vi "Main.vi"(7 "sweep rate, /min":dbl=0.2, 8 "sweep to:":dbl=4.0, 9 "sweep":T8(radio)=enum."2636a_smub") -> ()   [LabVIEW 2021] (continued)
                      n3296 = local read "SR830 1 addr"() -> (w4460:u8)
                      n3297 = Number To Decimal String(number=w4460) -> (decimal integer string=w4459:string)  [unwired: 1 in]
                      n3298 = GPIB Write(0:w4459, 1:"OUTR?1") -> (6:w4465:errorcluster)  [unwired: 3 in, 1 out]
                      n3299 = GPIB Read(0:w4459, 1:3200, 3:w4465) -> (5:w4463:string)  [unwired: 2 in, 2 out]
                      n3300 = Fract/Exp String To Number(string=w4463) -> (number=w4462:dbl)  [unwired: 3 in, 1 out]
                      n3301 = Build Array (concatenate)(w4467, w4462) -> (w4466:dbl[])
                    }
                  }
                  n3302 = property on="data" class="Arr (strict)"("Value"=w4457) -> ()  [unwired: 2 in, 2 out]
                }
                frame #1 {
                  # "check if out-of-phase\nsignal on lock-in 1 \nis to be measured"
                  n3303 = property on="data" class="Arr (strict)"() -> ("Value"=w4469:dbl[])  [unwired: 2 in, 2 out]
                  n3304 = local read "SR830 1 oop"() -> (w4468:bool)
                  n3305 = case shown="True" w4468 {
                    tunnel: w4469 -> [w4471 w4480]
                    tunnel: [w4471 w4479] -> w4470
                    frame False {
                      # "we are not measuring out of phase signal on lock-in 1 (SR830_1_oop)"
                    }
                    frame True {
                      # "we are  measuring lock-in 1, out of phase (SR830_1_oop)"
                      n3306 = local read "SR830 1 addr"() -> (w4473:u8)
                      n3307 = Number To Decimal String(number=w4473) -> (decimal integer string=w4472:string)  [unwired: 1 in]
                      n3308 = GPIB Write(0:w4472, 1:"OUTR?2") -> (6:w4478:errorcluster)  [unwired: 3 in, 1 out]
                      n3309 = GPIB Read(0:w4472, 1:3200, 3:w4478) -> (5:w4476:string)  [unwired: 2 in, 2 out]
                      n3310 = Fract/Exp String To Number(string=w4476) -> (number=w4475:dbl)  [unwired: 3 in, 1 out]
                      n3311 = Build Array (concatenate)(w4480, w4475) -> (w4479:dbl[])
                    }
                  }
                  n3312 = property on="data" class="Arr (strict)"("Value"=w4470) -> ()  [unwired: 2 in, 2 out]
                }
                frame #2 {
                  # "check if in-phase\nsignal on lock-in 2 \nis to be measured"
                  n3313 = property on="data" class="Arr (strict)"() -> ("Value"=w4482:dbl[])  [unwired: 2 in, 2 out]
                  n3314 = local read "SR830 2 ip"() -> (w4481:bool)
                  n3315 = case shown="True" w4481 {
                    tunnel: w4482 -> [w4484 w4493]
                    tunnel: [w4484 w4492] -> w4483
                    frame False {
                      # "we are not measuring in phase signal on lock-in 2 (SR830_2_ip)"
                    }
                    frame True {
                      # "we are  measuring lock-in 2, in phase (SR830_2_ip)"
                      n3316 = local read "SR830 2 addr"() -> (w4486:u8)
                      n3317 = Number To Decimal String(number=w4486) -> (decimal integer string=w4485:string)  [unwired: 1 in]
                      n3318 = GPIB Write(0:w4485, 1:"OUTP?1") -> (6:w4491:errorcluster)  [unwired: 3 in, 1 out]
                      n3319 = GPIB Read(0:w4485, 1:3200, 3:w4491) -> (5:w4489:string)  [unwired: 2 in, 2 out]
                      n3320 = Fract/Exp String To Number(string=w4489) -> (number=w4488:dbl)  [unwired: 3 in, 1 out]
                      n3321 = Build Array (concatenate)(w4493, w4488) -> (w4492:dbl[])
                    }
                  }
                  n3322 = property on="data" class="Arr (strict)"("Value"=w4483) -> ()  [unwired: 2 in, 2 out]
                }
                frame #3 {
                  # "check if out-of-phase\nsignal on lock-in 2 \nis to be measured"
                  n3323 = property on="data" class="Arr (strict)"() -> ("Value"=w4495:dbl[])  [unwired: 2 in, 2 out]
                  n3324 = local read "SR830 2 oop"() -> (w4494:bool)
                  n3325 = case shown="True" w4494 {
                    tunnel: w4495 -> [w4497 w4506]
                    tunnel: [w4497 w4505] -> w4496
                    frame False {
                      # "we are not measuring out of phase signal on lock-in 2 (SR830_2_oop)"
                    }
                    frame True {
                      # "we are  measuring lock-in 2, out of phase (SR830_2_oop)"
                      n3326 = local read "SR830 2 addr"() -> (w4499:u8)
                      n3327 = Number To Decimal String(number=w4499) -> (decimal integer string=w4498:string)  [unwired: 1 in]
                      n3328 = GPIB Write(0:w4498, 1:"OUTP?2") -> (6:w4504:errorcluster)  [unwired: 3 in, 1 out]
                      n3329 = GPIB Read(0:w4498, 1:3200, 3:w4504) -> (5:w4502:string)  [unwired: 2 in, 2 out]
                      n3330 = Fract/Exp String To Number(string=w4502) -> (number=w4501:dbl)  [unwired: 3 in, 1 out]
                      n3331 = Build Array (concatenate)(w4506, w4501) -> (w4505:dbl[])
                    }
                  }
                  n3332 = property on="data" class="Arr (strict)"("Value"=w4496) -> ()  [unwired: 2 in, 2 out]
                }
                frame #4 {
                  # "check if in-phase\nsignal on lock-in 3 \nis to be measured"
                  n3333 = property on="data" class="Arr (strict)"() -> ("Value"=w4508:dbl[])  [unwired: 2 in, 2 out]
                  n3334 = local read "SR830 3 ip"() -> (w4507:bool)
                  n3335 = case shown="True" w4507 {
                    tunnel: w4508 -> [w4510 w4519]
                    tunnel: [w4510 w4518] -> w4509
                    frame False {
                      # "we are not measuring in phase signal on lock-in 3 (SR830_3_ip)"
                    }
                    frame True {
                      # "we are  measuring lock-in 3, in phase (SR830_3_ip)"
                      n3336 = local read "SR830 3 addr"() -> (w4512:u8)
                      n3337 = Number To Decimal String(number=w4512) -> (decimal integer string=w4511:string)  [unwired: 1 in]
                      n3338 = GPIB Write(0:w4511, 1:"OUTP?1") -> (6:w4517:errorcluster)  [unwired: 3 in, 1 out]
                      n3339 = GPIB Read(0:w4511, 1:3200, 3:w4517) -> (5:w4515:string)  [unwired: 2 in, 2 out]
                      n3340 = Fract/Exp String To Number(string=w4515) -> (number=w4514:dbl)  [unwired: 3 in, 1 out]
                      n3341 = Build Array (concatenate)(w4519, w4514) -> (w4518:dbl[])
                    }
                  }
                  n3342 = property on="data" class="Arr (strict)"("Value"=w4509) -> ()  [unwired: 2 in, 2 out]
                }
                frame #5 {
                  # "check if out-of-phase\nsignal on lock-in 3 \nis to be measured"
                  n3343 = property on="data" class="Arr (strict)"() -> ("Value"=w4521:dbl[])  [unwired: 2 in, 2 out]
                  n3344 = local read "SR830 3 oop"() -> (w4520:bool)
                  n3345 = case shown="True" w4520 {
                    tunnel: w4521 -> [w4523 w4532]
                    tunnel: [w4523 w4531] -> w4522
                    frame False {
                      # "we are not measuring out of phase signal on lock-in 3 (SR830_3_oop)"
                    }
                    frame True {
                      # "we are  measuring lock-in 3, out of phase (SR830_3_oop)"
                      n3346 = local read "SR830 3 addr"() -> (w4525:u8)
                      n3347 = Number To Decimal String(number=w4525) -> (decimal integer string=w4524:string)  [unwired: 1 in]
                      n3348 = GPIB Write(0:w4524, 1:"OUTP?2") -> (6:w4530:errorcluster)  [unwired: 3 in, 1 out]
                      n3349 = GPIB Read(0:w4524, 1:3200, 3:w4530) -> (5:w4528:string)  [unwired: 2 in, 2 out]
                      n3350 = Fract/Exp String To Number(string=w4528) -> (number=w4527:dbl)  [unwired: 3 in, 1 out]
                      n3351 = Build Array (concatenate)(w4532, w4527) -> (w4531:dbl[])
                    }
                  }
                  n3352 = property on="data" class="Arr (strict)"("Value"=w4522) -> ()  [unwired: 2 in, 2 out]
                }
                frame #6 {
                  # "check if in-phase\nsignal on lock-in 4 \nis to be measured"
                  n3353 = property on="data" class="Arr (strict)"() -> ("Value"=w4534:dbl[])  [unwired: 2 in, 2 out]
                  n3354 = local read "SR830 4 ip"() -> (w4533:bool)
                  n3355 = case shown="True" w4533 {
                    tunnel: w4534 -> [w4536 w4545]
                    tunnel: [w4536 w4544] -> w4535
                    frame False {
                      # "we are not measuring in phase signal on lock-in 4 (SR830_4_ip)"
                    }
                    frame True {
                      # "we are  measuring lock-in 4, in phase (SR830_4_ip)"
                      n3356 = local read "SR830 4 addr"() -> (w4538:u8)
                      n3357 = Number To Decimal String(number=w4538) -> (decimal integer string=w4537:string)  [unwired: 1 in]
                      n3358 = GPIB Write(0:w4537, 1:"OUTP?1") -> (6:w4543:errorcluster)  [unwired: 3 in, 1 out]
                      n3359 = GPIB Read(0:w4537, 1:3200, 3:w4543) -> (5:w4541:string)  [unwired: 2 in, 2 out]
                      n3360 = Fract/Exp String To Number(string=w4541) -> (number=w4540:dbl)  [unwired: 3 in, 1 out]
                      n3361 = Build Array (concatenate)(w4545, w4540) -> (w4544:dbl[])
                    }
                  }
                  n3362 = property on="data" class="Arr (strict)"("Value"=w4535) -> ()  [unwired: 2 in, 2 out]
                }
                frame #7 {
                  # "check if out-of-phase\nsignal on lock-in 4 \nis to be measured"
                  n3363 = property on="data" class="Arr (strict)"() -> ("Value"=w4547:dbl[])  [unwired: 2 in, 2 out]
                  n3364 = local read "SR830 4 oop"() -> (w4546:bool)
                  n3365 = case shown="True" w4546 {
                    tunnel: w4547 -> [w4549 w4558]
                    tunnel: [w4549 w4557] -> w4548
                    frame False {
                      # "we are not measuring out of phase signal on lock-in 4 (SR830_4_oop)"
                    }
                    frame True {
                      # "we are  measuring lock-in 4, out of phase (SR830_4_oop)"
                      n3366 = local read "SR830 4 addr"() -> (w4551:u8)
                      n3367 = Number To Decimal String(number=w4551) -> (decimal integer string=w4550:string)  [unwired: 1 in]
                      n3368 = GPIB Write(0:w4550, 1:"OUTP?2") -> (6:w4556:errorcluster)  [unwired: 3 in, 1 out]
                      n3369 = GPIB Read(0:w4550, 1:3200, 3:w4556) -> (5:w4554:string)  [unwired: 2 in, 2 out]
                      n3370 = Fract/Exp String To Number(string=w4554) -> (number=w4553:dbl)  [unwired: 3 in, 1 out]
                      n3371 = Build Array (concatenate)(w4558, w4553) -> (w4557:dbl[])
                    }
                  }
                  n3372 = property on="data" class="Arr (strict)"("Value"=w4548) -> ()  [unwired: 2 in, 2 out]
                }
                frame #8 {
                  n3373 = property on="data" class="Arr (strict)"() -> ("Value"=w4560:dbl[])  [unwired: 2 in, 2 out]
                  n3374 = local read "SR830 5 ip"() -> (w4559:bool)
                  n3375 = case shown="True" w4559 {
                    tunnel: w4560 -> [w4562 w4571]
                    tunnel: [w4562 w4570] -> w4561
                    frame False {
                    }
                    frame True {
                      n3376 = local read "SR830 5 addr"() -> (w4564:u8)
                      n3377 = Number To Decimal String(number=w4564) -> (decimal integer string=w4563:string)  [unwired: 1 in]
                      n3378 = GPIB Write(0:w4563, 1:"OUTP?1") -> (6:w4569:errorcluster)  [unwired: 3 in, 1 out]
                      n3379 = GPIB Read(0:w4563, 1:3200, 3:w4569) -> (5:w4567:string)  [unwired: 2 in, 2 out]
                      n3380 = Fract/Exp String To Number(string=w4567) -> (number=w4566:dbl)  [unwired: 3 in, 1 out]
                      n3381 = Build Array (concatenate)(w4571, w4566) -> (w4570:dbl[])
                    }
                  }
                  n3382 = property on="data" class="Arr (strict)"("Value"=w4561) -> ()  [unwired: 2 in, 2 out]
                }
                frame #9 {
                  n3383 = property on="data" class="Arr (strict)"() -> ("Value"=w4573:dbl[])  [unwired: 2 in, 2 out]
                  n3384 = local read "SR830 5 oop"() -> (w4572:bool)
                  n3385 = case shown="True" w4572 {
                    tunnel: w4573 -> [w4575 w4584]
                    tunnel: [w4575 w4583] -> w4574
                    frame False {
                    }
                    frame True {
                      n3386 = local read "SR830 5 addr"() -> (w4577:u8)
                      n3387 = Number To Decimal String(number=w4577) -> (decimal integer string=w4576:string)  [unwired: 1 in]
                      n3388 = GPIB Write(0:w4576, 1:"OUTP?2") -> (6:w4582:errorcluster)  [unwired: 3 in, 1 out]
                      n3389 = GPIB Read(0:w4576, 1:3200, 3:w4582) -> (5:w4580:string)  [unwired: 2 in, 2 out]
                      n3390 = Fract/Exp String To Number(string=w4580) -> (number=w4579:dbl)  [unwired: 3 in, 1 out]
                      n3391 = Build Array (concatenate)(w4584, w4579) -> (w4583:dbl[])
                    }
                  }
                  n3392 = property on="data" class="Arr (strict)"("Value"=w4574) -> ()  [unwired: 2 in, 2 out]
                }
                frame #10 {
                  # "check if voltage \non 2400 SouceMeter 1\nis to be measured"
                  n3393 = property on="data" class="Arr (strict)"() -> ("Value"=w4586:dbl[])  [unwired: 2 in, 2 out]
                  n3394 = local read "2400 1 meas v"() -> (w4585:bool)
                  n3395 = case shown="True" w4585 {
                    tunnel: w4586 -> [w4588 w4599]
                    tunnel: [w4588 w4598] -> w4587
                    frame False {
                      # "we are not measuring 2400 1, voltage (2400_1_v)"
                    }
                    frame True {
                      # "we are  measuring 2400 1, voltage (2400_1_v)"
                      n3396 = local read "2400 1 addr"() -> (w4593:u8)
                      n3397 = Number To Decimal String(number=w4593) -> (decimal integer string=w4592:string)  [unwired: 1 in]
                      n3398 = GPIB Write(0:w4592, 1:":READ?") -> (6:w4597:errorcluster)  [unwired: 3 in, 1 out]
                      n3399 = GPIB Read(0:w4592, 1:3200, 3:w4597) -> (5:w4590:string)  [unwired: 2 in, 2 out]
                      n3400 = String Subset(string=w4590, length (rest)=13) -> (substring=w4589:string)  [unwired: 1 in]
                      n3401 = Fract/Exp String To Number(string=w4589) -> (number=w4595:dbl)  [unwired: 3 in, 1 out]
                      n3402 = Build Array (concatenate)(w4599, w4595) -> (w4598:dbl[])
                    }
                  }
                  n3403 = property on="data" class="Arr (strict)"("Value"=w4587) -> ()  [unwired: 2 in, 2 out]
                }
                frame #11 {
                  # "check if current \non 2400 SouceMeter 1\nis to be measured"
                  n3404 = property on="data" class="Arr (strict)"() -> ("Value"=w4601:dbl[])  [unwired: 2 in, 2 out]
                  n3405 = local read "2400 1 meas i"() -> (w4600:bool)
                  n3406 = case shown="True" w4600 {
                    tunnel: w4601 -> [w4603 w4615]
                    tunnel: [w4603 w4614] -> w4602
                    frame False {
                      # "we are not measuring 2400 1, current (2400_1_i)"
                    }
                    frame True {
                      # "we are  measuring 2400 1, current (2400_1_i)"
                      n3407 = local read "2400 1 addr"() -> (w4609:u8)
                      n3408 = Number To Decimal String(number=w4609) -> (decimal integer string=w4608:string)  [unwired: 1 in]
                      n3409 = GPIB Write(0:w4608, 1:":READ?") -> (6:w4613:errorcluster)  [unwired: 3 in, 1 out]
                      n3410 = GPIB Read(0:w4608, 1:3200, 3:w4613) -> (5:w4606:string)  [unwired: 2 in, 2 out]
                      n3411 = String Subset(string=w4606, offset (0)=14, length (rest)=13) -> (substring=w4605:string)
                      n3412 = Fract/Exp String To Number(string=w4605) -> (number=w4611:dbl)  [unwired: 3 in, 1 out]
                      n3413 = Build Array (concatenate)(w4615, w4611) -> (w4614:dbl[])
                    }
                  }
                  n3414 = property on="data" class="Arr (strict)"("Value"=w4602) -> ()  [unwired: 2 in, 2 out]
                }
                frame #12 {
                  # "check if voltage \non 2400 SouceMeter 2\nis to be measured"
                  n3415 = property on="data" class="Arr (strict)"() -> ("Value"=w4617:dbl[])  [unwired: 2 in, 2 out]
                  n3416 = local read "2400 2 meas v"() -> (w4616:bool)
                  n3417 = case shown="True" w4616 {
                    tunnel: w4617 -> [w4619 w4630]
                    tunnel: [w4619 w4629] -> w4618
                    frame False {
                      # "we are not measuring 2400 2, voltage (2400_2_v)"
                    }
                    frame True {
                      # "we are  measuring 2400 2, voltage (2400_2_v)"
                      n3418 = local read "2400 2 addr"() -> (w4624:u8)
                      n3419 = Number To Decimal String(number=w4624) -> (decimal integer string=w4623:string)  [unwired: 1 in]
                      n3420 = GPIB Write(0:w4623, 1:":READ?") -> (6:w4628:errorcluster)  [unwired: 3 in, 1 out]
                      n3421 = GPIB Read(0:w4623, 1:3200, 3:w4628) -> (5:w4621:string)  [unwired: 2 in, 2 out]
                      n3422 = String Subset(string=w4621, length (rest)=13) -> (substring=w4620:string)  [unwired: 1 in]
                      n3423 = Fract/Exp String To Number(string=w4620) -> (number=w4626:dbl)  [unwired: 3 in, 1 out]
                      n3424 = Build Array (concatenate)(w4630, w4626) -> (w4629:dbl[])
                    }
                  }
                  n3425 = property on="data" class="Arr (strict)"("Value"=w4618) -> ()  [unwired: 2 in, 2 out]
                }
                frame #13 {
                  # "check if current \non 2400 SouceMeter 2\nis to be measured"
                  n3426 = property on="data" class="Arr (strict)"() -> ("Value"=w4632:dbl[])  [unwired: 2 in, 2 out]
                  n3427 = local read "2400 2 meas i"() -> (w4631:bool)
                  n3428 = case shown="True" w4631 {
                    tunnel: w4632 -> [w4634 w4646]
                    tunnel: [w4634 w4645] -> w4633
                    frame False {
                      # "we are not measuring 2400 2, current (2400_2_i)"
                    }
                    frame True {
                      # "we are  measuring 2400 2, current (2400_2_i)"
                      n3429 = local read "2400 2 addr"() -> (w4640:u8)
                      n3430 = Number To Decimal String(number=w4640) -> (decimal integer string=w4639:string)  [unwired: 1 in]
                      n3431 = GPIB Write(0:w4639, 1:":READ?") -> (6:w4644:errorcluster)  [unwired: 3 in, 1 out]
                      n3432 = GPIB Read(0:w4639, 1:3200, 3:w4644) -> (5:w4637:string)  [unwired: 2 in, 2 out]
                      n3433 = String Subset(string=w4637, offset (0)=14, length (rest)=13) -> (substring=w4636:string)
                      n3434 = Fract/Exp String To Number(string=w4636) -> (number=w4642:dbl)  [unwired: 3 in, 1 out]
                      n3435 = Build Array (concatenate)(w4646, w4642) -> (w4645:dbl[])
                    }
                  }
                  n3436 = property on="data" class="Arr (strict)"("Value"=w4633) -> ()  [unwired: 2 in, 2 out]
                }
                frame #14 {
                  # "check if voltage \non 2400 SouceMeter 3\nis to be measured"
                  n3437 = property on="data" class="Arr (strict)"() -> ("Value"=w4648:dbl[])  [unwired: 2 in, 2 out]
                  n3438 = local read "2400 3 meas v"() -> (w4647:bool)
                  n3439 = case shown="True" w4647 {
                    tunnel: w4648 -> [w4650 w4661]
                    tunnel: [w4650 w4660] -> w4649
                    frame False {
                      # "we are not measuring 2400 3, voltage (2400_3_v)"
                    }
                    frame True {
                      # "we are  measuring 2400 3, voltage (2400_3_v)"
                      n3440 = local read "2400 3 addr"() -> (w4655:u8)
                      n3441 = Number To Decimal String(number=w4655) -> (decimal integer string=w4654:string)  [unwired: 1 in]
                      n3442 = GPIB Write(0:w4654, 1:":READ?") -> (6:w4659:errorcluster)  [unwired: 3 in, 1 out]
                      n3443 = GPIB Read(0:w4654, 1:3200, 3:w4659) -> (5:w4652:string)  [unwired: 2 in, 2 out]
                      n3444 = String Subset(string=w4652, length (rest)=13) -> (substring=w4651:string)  [unwired: 1 in]
                      n3445 = Fract/Exp String To Number(string=w4651) -> (number=w4657:dbl)  [unwired: 3 in, 1 out]
                      n3446 = Build Array (concatenate)(w4661, w4657) -> (w4660:dbl[])
                    }
                  }
                  n3447 = property on="data" class="Arr (strict)"("Value"=w4649) -> ()  [unwired: 2 in, 2 out]
                }
                frame #15 {
                  # "check if current \non 2400 SouceMeter 3\nis to be measured"
                  n3448 = property on="data" class="Arr (strict)"() -> ("Value"=w4663:dbl[])  [unwired: 2 in, 2 out]
                  n3449 = local read "2400 3 meas i"() -> (w4662:bool)
                  n3450 = case shown="True" w4662 {
                    tunnel: w4663 -> [w4665 w4677]
                    tunnel: [w4665 w4676] -> w4664
                    frame False {
                      # "we are not measuring 2400 3, current (2400_3_i)"
                    }
                    frame True {
                      # "we are  measuring 2400 3, current (2400_3_i)"
                      n3451 = local read "2400 3 addr"() -> (w4671:u8)
                      n3452 = Number To Decimal String(number=w4671) -> (decimal integer string=w4670:string)  [unwired: 1 in]
                      n3453 = GPIB Write(0:w4670, 1:":READ?") -> (6:w4675:errorcluster)  [unwired: 3 in, 1 out]
                      n3454 = GPIB Read(0:w4670, 1:3200, 3:w4675) -> (5:w4668:string)  [unwired: 2 in, 2 out]
                      n3455 = String Subset(string=w4668, offset (0)=14, length (rest)=13) -> (substring=w4667:string)
                      n3456 = Fract/Exp String To Number(string=w4667) -> (number=w4673:dbl)  [unwired: 3 in, 1 out]
                      n3457 = Build Array (concatenate)(w4677, w4673) -> (w4676:dbl[])
                    }
                  }
                  n3458 = property on="data" class="Arr (strict)"("Value"=w4664) -> ()  [unwired: 2 in, 2 out]
                }
                frame #16 {
                  # "check if 1st channel \non Keithley 2182A 1\nis to be measured"
                  n3459 = property on="data" class="Arr (strict)"() -> ("Value"=w4679:dbl[])  [unwired: 2 in, 2 out]
                  n3460 = local read "2182A 1 ch1"() -> (w4678:bool)
                  n3461 = case shown="True" w4678 {
                    tunnel: w4679 -> [w4681 w4690]
                    tunnel: [w4681 w4689] -> w4680
                    frame False {
                      # "we are not measuring 2182A 1 channel 1 (2182A_1_ch1)"
                    }
                    frame True {
                      # "we are  measuring 2182A 1 channel 1 (2182A_1_ch1)"
                      n3462 = local read "2182A 1 addr"() -> (w4684:u8)
                      n3463 = Number To Decimal String(number=w4684) -> (decimal integer string=w4683:string)  [unwired: 1 in]
                      n3464 = GPIB Write(0:w4683, 1:":SENSe:DATA:FRES?") -> (6:w4688:errorcluster)  [unwired: 3 in, 1 out]
                      n3465 = GPIB Read(0:w4683, 1:200, 3:w4688) -> (5:w4682:string)  [unwired: 2 in, 2 out]
                      n3466 = Fract/Exp String To Number(string=w4682) -> (number=w4686:dbl)  [unwired: 3 in, 1 out]
                      n3467 = Build Array (concatenate)(w4690, w4686) -> (w4689:dbl[])
                    }
                  }
                  n3468 = property on="data" class="Arr (strict)"("Value"=w4680) -> ()  [unwired: 2 in, 2 out]
                }
                frame #17 {
                  # "check if 2nd channel \non Keithley 2182A 1\nis to be measured"
                  n3469 = property on="data" class="Arr (strict)"() -> ("Value"=w4692:dbl[])  [unwired: 2 in, 2 out]
                  n3470 = local read "2182A 1 ch2"() -> (w4691:bool)
                  n3471 = case shown="True" w4691 {
                    tunnel: w4692 -> [w4694 w4707]
                    tunnel: [w4694 w4706] -> w4693
                    frame False {
                      # "we are not measuring 2182A 1 channel 2 (2182A_1_ch2)"
                    }
                    frame True {
                      # "switching to channel 2 and then\nback to channel 1"
                      # "we are  measuring 2182A 1 channel 2 (2182A_1_ch2)"
                      n3472 = local read "2182A 1 addr"() -> (w4701:u8)
                      n3473 = Number To Decimal String(number=w4701) -> (decimal integer string=w4696:string)  [unwired: 1 in]
                      n3474 = GPIB Write(0:w4696, 1:":SENSe:CHAN 2") -> (6:w4698:errorcluster)  [unwired: 3 in, 1 out]
                      n3475 = GPIB Write(0:w4696, 1:":SENSe:DATA:FRES?", 3:w4698) -> (6:w4705:errorcluster)  [unwired: 2 in, 1 out]
                      n3476 = GPIB Read(0:w4696, 1:200, 3:w4705) -> (5:w4700:string, 7:w4697:errorcluster)  [unwired: 2 in, 1 out]
                      n3477 = GPIB Write(0:w4696, 1:":SENSe:CHAN 1", 3:w4697) -> ()  [unwired: 2 in, 2 out]
                      n3478 = Fract/Exp String To Number(string=w4700) -> (number=w4703:dbl)  [unwired: 3 in, 1 out]
                      n3479 = Build Array (concatenate)(w4707, w4703) -> (w4706:dbl[])
                    }
                  }
                  n3480 = property on="data" class="Arr (strict)"("Value"=w4693) -> ()  [unwired: 2 in, 2 out]
                }
                frame #18 {
                  # "check if 1st channel \non Keithley 2182A 2\nis to be measured"
                  n3481 = property on="data" class="Arr (strict)"() -> ("Value"=w4709:dbl[])  [unwired: 2 in, 2 out]
                  n3482 = local read "2182A 2 ch1"() -> (w4708:bool)
                  n3483 = case shown="True" w4708 {
                    tunnel: w4709 -> [w4711 w4720]
                    tunnel: [w4711 w4719] -> w4710
                    frame False {
                      # "we are not measuring 2182A 2 channel 1 (2182A_2_ch1)"
                    }
                    frame True {
                      # "we are  measuring 2182A 2 channel 1 (2182A_2_ch1)"
                      n3484 = local read "2182A 2 addr"() -> (w4714:u8)
                      n3485 = Number To Decimal String(number=w4714) -> (decimal integer string=w4713:string)  [unwired: 1 in]
                      n3486 = GPIB Write(0:w4713, 1:":SENSe:DATA:FRES?") -> (6:w4718:errorcluster)  [unwired: 3 in, 1 out]
                      n3487 = GPIB Read(0:w4713, 1:200, 3:w4718) -> (5:w4712:string)  [unwired: 2 in, 2 out]
                      n3488 = Fract/Exp String To Number(string=w4712) -> (number=w4716:dbl)  [unwired: 3 in, 1 out]
                      n3489 = Build Array (concatenate)(w4720, w4716) -> (w4719:dbl[])
                    }
                  }
                  n3490 = property on="data" class="Arr (strict)"("Value"=w4710) -> ()  [unwired: 2 in, 2 out]
                }
                frame #19 {
                  # "check if 2nd channel \non Keithley 2182A 2\nis to be measured"
                  n3491 = property on="data" class="Arr (strict)"() -> ("Value"=w4722:dbl[])  [unwired: 2 in, 2 out]
                  n3492 = local read "2182A 2 ch2"() -> (w4721:bool)
                  n3493 = case shown="True" w4721 {
                    tunnel: w4722 -> [w4724 w4737]
                    tunnel: [w4724 w4736] -> w4723
                    frame False {
                      # "we are not measuring 2182A 2 channel 2 (2182A_2_ch2)"
                    }
                    frame True {
                      # "switching to channel 2 and then\nback to channel 1"
                      # "we are  measuring 2182A 2 channel 2 (2182A_2_ch2)"
                      n3494 = local read "2182A 2 addr"() -> (w4731:u8)
                      n3495 = Number To Decimal String(number=w4731) -> (decimal integer string=w4726:string)  [unwired: 1 in]
                      n3496 = GPIB Write(0:w4726, 1:":SENSe:CHAN 2") -> (6:w4728:errorcluster)  [unwired: 3 in, 1 out]
                      n3497 = GPIB Write(0:w4726, 1:":SENSe:DATA:FRES?", 3:w4728) -> (6:w4735:errorcluster)  [unwired: 2 in, 1 out]
                      n3498 = GPIB Read(0:w4726, 1:200, 3:w4735) -> (5:w4730:string, 7:w4727:errorcluster)  [unwired: 2 in, 1 out]
                      n3499 = GPIB Write(0:w4726, 1:":SENSe:CHAN 1", 3:w4727) -> ()  [unwired: 2 in, 2 out]
                      n3500 = Fract/Exp String To Number(string=w4730) -> (number=w4733:dbl)  [unwired: 3 in, 1 out]
                      n3501 = Build Array (concatenate)(w4737, w4733) -> (w4736:dbl[])
                    }
                  }
                  n3502 = property on="data" class="Arr (strict)"("Value"=w4723) -> ()  [unwired: 2 in, 2 out]
                }
                frame #20 {
                  # "check if 1st channel \non Keithley 2182A 3\nis to be measured"
                  n3503 = property on="data" class="Arr (strict)"() -> ("Value"=w4739:dbl[])  [unwired: 2 in, 2 out]
                  n3504 = local read "2182A 3 ch1"() -> (w4738:bool)
                  n3505 = case shown="True" w4738 {
                    tunnel: w4739 -> [w4741 w4750]
                    tunnel: [w4741 w4749] -> w4740
                    frame False {
                      # "we are not measuring 2182A 3 channel 1 (2182A_3_ch1)"
                    }
                    frame True {
                      # "we are  measuring 2182A 3 channel 1 (2182A_3_ch1)"
                      n3506 = local read "2182A 3 addr"() -> (w4744:u8)
                      n3507 = Number To Decimal String(number=w4744) -> (decimal integer string=w4743:string)  [unwired: 1 in]
                      n3508 = GPIB Write(0:w4743, 1:":SENSe:DATA:FRES?") -> (6:w4748:errorcluster)  [unwired: 3 in, 1 out]
                      n3509 = GPIB Read(0:w4743, 1:200, 3:w4748) -> (5:w4742:string)  [unwired: 2 in, 2 out]
                      n3510 = Fract/Exp String To Number(string=w4742) -> (number=w4746:dbl)  [unwired: 3 in, 1 out]
                      n3511 = Build Array (concatenate)(w4750, w4746) -> (w4749:dbl[])
                    }
                  }
                  n3512 = property on="data" class="Arr (strict)"("Value"=w4740) -> ()  [unwired: 2 in, 2 out]
                }
                frame #21 {
                  # "check if 2nd channel \non Keithley 2182A 3\nis to be measured"
                  n3513 = property on="data" class="Arr (strict)"() -> ("Value"=w4752:dbl[])  [unwired: 2 in, 2 out]
                  n3514 = local read "2182A 3 ch2"() -> (w4751:bool)
                  n3515 = case shown="True" w4751 {
                    tunnel: w4752 -> [w4754 w4767]
                    tunnel: [w4754 w4766] -> w4753
                    frame False {
                      # "we are not measuring 2182A 3 channel 2 (2182A_3_ch2)"
                    }
                    frame True {
                      # "switching to channel 2 and then\nback to channel 1"
                      # "we are  measuring 2182A 3 channel 2 (2182A_3_ch2)"
                      n3516 = local read "2182A 3 addr"() -> (w4761:u8)
                      n3517 = Number To Decimal String(number=w4761) -> (decimal integer string=w4756:string)  [unwired: 1 in]
                      n3518 = GPIB Write(0:w4756, 1:":SENSe:CHAN 2") -> (6:w4758:errorcluster)  [unwired: 3 in, 1 out]
                      n3519 = GPIB Write(0:w4756, 1:":SENSe:DATA:FRES?", 3:w4758) -> (6:w4765:errorcluster)  [unwired: 2 in, 1 out]
                      n3520 = GPIB Read(0:w4756, 1:200, 3:w4765) -> (5:w4760:string, 7:w4757:errorcluster)  [unwired: 2 in, 1 out]
                      n3521 = GPIB Write(0:w4756, 1:":SENSe:CHAN 1", 3:w4757) -> ()  [unwired: 2 in, 2 out]
                      n3522 = Fract/Exp String To Number(string=w4760) -> (number=w4763:dbl)  [unwired: 3 in, 1 out]
                      n3523 = Build Array (concatenate)(w4767, w4763) -> (w4766:dbl[])
                    }
                  }
                  n3524 = property on="data" class="Arr (strict)"("Value"=w4753) -> ()  [unwired: 2 in, 2 out]
                }
                frame #22 {
                  # "check if 1st channel \non Keithley 2182A 4\nis to be measured"
                  n3525 = property on="data" class="Arr (strict)"() -> ("Value"=w4769:dbl[])  [unwired: 2 in, 2 out]
                  n3526 = local read "2182A 4 ch1"() -> (w4768:bool)
                  n3527 = case shown="True" w4768 {
                    tunnel: w4769 -> [w4771 w4780]
                    tunnel: [w4771 w4779] -> w4770
                    frame False {
                      # "we are not measuring 2182A 4 channel 1 (2182A_4_ch1)"
                    }
                    frame True {
                      # "we are  measuring 2182A 4 channel 1 (2182A_4_ch1)"
                      n3528 = local read "2182A 4 addr"() -> (w4774:u8)
                      n3529 = Number To Decimal String(number=w4774) -> (decimal integer string=w4773:string)  [unwired: 1 in]
                      n3530 = GPIB Write(0:w4773, 1:":SENSe:DATA:FRES?") -> (6:w4778:errorcluster)  [unwired: 3 in, 1 out]
                      n3531 = GPIB Read(0:w4773, 1:200, 3:w4778) -> (5:w4772:string)  [unwired: 2 in, 2 out]
                      n3532 = Fract/Exp String To Number(string=w4772) -> (number=w4776:dbl)  [unwired: 3 in, 1 out]
                      n3533 = Build Array (concatenate)(w4780, w4776) -> (w4779:dbl[])
                    }
                  }
                  n3534 = property on="data" class="Arr (strict)"("Value"=w4770) -> ()  [unwired: 2 in, 2 out]
                }
                frame #23 {
                  # "check if 2nd channel \non Keithley 2182A 4\nis to be measured"
                  n3535 = property on="data" class="Arr (strict)"() -> ("Value"=w4782:dbl[])  [unwired: 2 in, 2 out]
                  n3536 = local read "2182A 4 ch2"() -> (w4781:bool)
                  n3537 = case shown="False" w4781 {
                    tunnel: w4782 -> [w4784 w4797]
                    tunnel: [w4784 w4796] -> w4783
                    frame False {
                      # "we are not measuring 2182A 4 channel 2 (2182A_4_ch2)"
                    }
                    frame True {
                      # "switching to channel 2 and then\nback to channel 1"
                      # "we are  measuring 2182A 4 channel 2 (2182A_4_ch2)"
                      n3538 = local read "2182A 4 addr"() -> (w4791:u8)
                      n3539 = Number To Decimal String(number=w4791) -> (decimal integer string=w4786:string)  [unwired: 1 in]
                      n3540 = GPIB Write(0:w4786, 1:":SENSe:CHAN 2") -> (6:w4788:errorcluster)  [unwired: 3 in, 1 out]
                      n3541 = GPIB Write(0:w4786, 1:":SENSe:DATA:FRES?", 3:w4788) -> (6:w4795:errorcluster)  [unwired: 2 in, 1 out]
                      n3542 = GPIB Read(0:w4786, 1:200, 3:w4795) -> (5:w4790:string, 7:w4787:errorcluster)  [unwired: 2 in, 1 out]
                      n3543 = GPIB Write(0:w4786, 1:":SENSe:CHAN 1", 3:w4787) -> ()  [unwired: 2 in, 2 out]
                      n3544 = Fract/Exp String To Number(string=w4790) -> (number=w4793:dbl)  [unwired: 3 in, 1 out]
                      n3545 = Build Array (concatenate)(w4797, w4793) -> (w4796:dbl[])
                    }
                  }
                  n3546 = property on="data" class="Arr (strict)"("Value"=w4783) -> ()  [unwired: 2 in, 2 out]
                }
                frame #24 {
                  # "check if voltage on\nKeithley 2636A smua\nis to be measured"
                  n3547 = local read "2636A smua meas v"() -> (w4798:bool)
                  n3548 = property on="data" class="Arr (strict)"() -> ("Value"=w4799:dbl[])  [unwired: 2 in, 2 out]
                  n3549 = case shown="True" w4798 {
                    tunnel: w4799 -> [w4801 w4807]
                    tunnel: [w4801 w4806] -> w4800
                    frame False {
                      # "we are not measuring voltage on 2636A smua (2636A_smua_v)"
                    }
                    frame True {
                      # "we are  measuring voltage on 2636A smua (2636A_smua_v)"
                      n3550 = local read "2614A addr"() -> (w4802:refnum<visa-resource-name>)
                      n3551 = call "SinglePointMeasurement.vi"("Measure"=Measure."Voltage", "Channel"=Channel."a", "VISA resource name 2"=w4802) -> ("Measuremet"=w4804:dbl)  [unwired: 3 in, 4 out]
                      n3552 = Build Array (concatenate)(w4807, w4804) -> (w4806:dbl[])
                    }
                  }
                  n3553 = property on="data" class="Arr (strict)"("Value"=w4800) -> ()  [unwired: 2 in, 2 out]
                }
                frame #25 {
                  # "check if current on\nKeithley 2636A smua\nis to be measured"
                  n3554 = local read "2636A smua meas i"() -> (w4808:bool)
                  n3555 = property on="data" class="Arr (strict)"() -> ("Value"=w4809:dbl[])  [unwired: 2 in, 2 out]
                  n3556 = case shown="True" w4808 {
                    tunnel: w4809 -> [w4811 w4814]
                    tunnel: [w4811 w4813] -> w4810
                    frame False {
                      # "we are not measuring current on 2636A smua (2636A_smua_i)"
                    }
                    frame True {
                      # "we are  measuring current on 2636A smua (2636A_smua_i)"
                      n3557 = stacked-sequence {
                        tunnel: [_ w4823] -> w4812
                        frame #0 {
                          n3558 = local read "auto\nrange A"() -> (w4818:bool)
                          n3559 = local read "2614A addr"() -> (w4821:refnum<visa-resource-name>)
                          n3560 = Select(t="smua.AUTORANGE_ON", s=w4818, f="smua.AUTORANGE_OFF") -> (s? t:f=w4816:string)
                          n3561 = Concatenate Strings("smua.measure.autorangei = ", w4816) -> (w4815:string)
                          n3562 = VISA Write(VISA resource name=w4821, write buffer=w4815) -> ()  [unwired: 1 in, 3 out]
                        }
                        frame #1 {
                          n3563 = local read "2614A addr"() -> (w4825:refnum<visa-resource-name>)
                          n3564 = call "SinglePointMeasurement.vi"("Measure"=Measure."Current", "Channel"=Channel."a", "VISA resource name 2"=w4825) -> ("Measuremet"=w4823:dbl)  [unwired: 3 in, 4 out]
                        }
                      }
                      n3565 = Build Array (concatenate)(w4814, w4812) -> (w4813:dbl[])
                    }
                  }
                  n3566 = property on="data" class="Arr (strict)"("Value"=w4810) -> ()  [unwired: 2 in, 2 out]
                }
                frame #26 {
                  # "check if voltage on\nKeithley 2636A smub\nis to be measured"
                  n3567 = local read "2636A smub meas v"() -> (w4826:bool)
                  n3568 = property on="data" class="Arr (strict)"() -> ("Value"=w4827:dbl[])  [unwired: 2 in, 2 out]
                  n3569 = case shown="True" w4826 {
                    tunnel: w4827 -> [w4829 w4835]
                    tunnel: [w4829 w4834] -> w4828
                    frame False {
                      # "we are not measuring voltage on 2636A smub (2636A_smub_v)"
                    }
                    frame True {
                      # "we are  measuring voltage on 2636A smub (2636A_smub_v)"
                      n3570 = local read "2614A addr"() -> (w4833:refnum<visa-resource-name>)
                      n3571 = call "SinglePointMeasurement.vi"("Measure"=Measure."Voltage", "Channel"=Channel."b", "VISA resource name 2"=w4833) -> ("Measuremet"=w4831:dbl)  [unwired: 3 in, 4 out]
                      n3572 = Build Array (concatenate)(w4835, w4831) -> (w4834:dbl[])
                    }
                  }
                  n3573 = property on="data" class="Arr (strict)"("Value"=w4828) -> ()  [unwired: 2 in, 2 out]
                }
                frame #27 {
                  # "check if current on\nKeithley 2636A smub\nis to be measured"
                  n3574 = local read "2636A smub meas i"() -> (w4836:bool)
                  n3575 = property on="data" class="Arr (strict)"() -> ("Value"=w4837:dbl[])  [unwired: 2 in, 2 out]
                  n3576 = case shown="True" w4836 {
                    tunnel: w4837 -> [w4839 w4842]
                    tunnel: [w4839 w4841] -> w4838
                    frame False {
                      # "we are not measuring current on 2636A smub (2636A_smub_i)"
                    }
                    frame True {
                      # "we are  measuring current on 2636A smub (2636A_smub_i)"
                      n3577 = stacked-sequence {
                        tunnel: [_ w4851] -> w4840
                        frame #0 {
                          n3578 = local read "auto\nrange B"() -> (w4846:bool)
                          n3579 = local read "2614A addr"() -> (w4849:refnum<visa-resource-name>)
                          n3580 = Select(t="smub.AUTORANGE_ON", s=w4846, f="smub.AUTORANGE_OFF") -> (s? t:f=w4844:string)
                          n3581 = Concatenate Strings("smub.measure.autorangei = ", w4844) -> (w4843:string)
                          n3582 = VISA Write(VISA resource name=w4849, write buffer=w4843) -> ()  [unwired: 1 in, 3 out]
                        }
                        frame #1 {
                          n3583 = local read "2614A addr"() -> (w4853:refnum<visa-resource-name>)
                          n3584 = call "SinglePointMeasurement.vi"("Measure"=Measure."Current", "Channel"=Channel."b", "VISA resource name 2"=w4853) -> ("Measuremet"=w4851:dbl)  [unwired: 3 in, 4 out]
                        }
                      }
                      n3585 = Build Array (concatenate)(w4842, w4840) -> (w4841:dbl[])
                    }
                  }
                  n3586 = property on="data" class="Arr (strict)"("Value"=w4838) -> ()  [unwired: 2 in, 2 out]
                }
                frame #28 {
                  # "check if time\nis to be measured"
                  n3587 = property on="data" class="Arr (strict)"() -> ("Value"=w4856:dbl[])  [unwired: 2 in, 2 out]
                  n3588 = local read "measure time"() -> (w4855:bool)
                  n3589 = case shown="True" w4855 {
                    tunnel: w4856 -> [w4858 w4864]
                    tunnel: [w4858 w4863] -> w4857
                    tunnel: w4854 -> [_ w4861]
                    frame False {
                      # "we are not measuring time"
                    }
                    frame True {
                      # "seconds from the beginning of month"
                      # "we are  measuring time"
                      n3590 = call "timeInSeconds.vi"() -> ("Numeric"=w4862:dbl, "current time"=w4859:timestamp)  [unwired: 2 in]
                      n3591 = property on="current time" class="AbsTime (strict)"("Value"=w4859) -> ()  [unwired: 2 in, 2 out]
                      n3592 = Subtract(x=w4862, y=w4861) -> (x-y=w4860:dbl)
                      n3593 = Build Array (concatenate)(w4864, w4860) -> (w4863:dbl[])
                    }
                  }
                  n3594 = property on="data" class="Arr (strict)"("Value"=w4857) -> ()  [unwired: 2 in, 2 out]
                }
                frame #29 {
                  n3595 = local read "MagnetField"() -> (w4865:bool)
                  n3596 = property on="data" class="Arr (strict)"() -> ("Value"=w4866:dbl[])  [unwired: 2 in, 2 out]
                  n3597 = case shown="True" w4865 {
                    tunnel: w4866 -> [w4868 w4871]
                    tunnel: [w4868 w4870] -> w4867
                    frame False {
                      # "we are not Measuring magnetic field on IPS120-0"
                    }
                    frame True {
                      # "Measure magnetic field on Teslatron_iPS_Field"
                      n3598 = call "TRITON_Read Field.vi"() -> ("Measurement"=w4869:dbl)  [unwired: 2 in, 1 out]
                      n3599 = Build Array (concatenate)(w4871, w4869) -> (w4870:dbl[])
                    }
                  }
                  n3600 = property on="data" class="Arr (strict)"("Value"=w4867) -> ()  [unwired: 2 in, 2 out]
                }
                frame #30 {
                  n3601 = property on="data" class="Arr (strict)"() -> ("Value"=w4873:dbl[])  [unwired: 2 in, 2 out]
                  n3602 = property on="Magnet_T" class="Bool (strict)"() -> ("Value"=w4872:bool)  [unwired: 2 in, 2 out]
                  n3603 = case shown="True" w4872 {
                    tunnel: w4873 -> [w4875 w4879]
                    tunnel: [w4875 w4878] -> w4874
                    frame False {
                      # "we are not Measuring magnetic field on IPS120-0"
                    }
                    frame True {
                      # "Measure magnetic_T on Teslatron"
                      n3604 = call "TRITON_Read Temperature.vi"("Channel"=13 ("Ch2")) -> ("Measuremet"=w4876:dbl)  [unwired: 1 in, 1 out]
                      n3605 = Build Array (concatenate)(w4879, w4876) -> (w4878:dbl[])
                    }
                  }
                  n3606 = property on="data" class="Arr (strict)"("Value"=w4874) -> ()  [unwired: 2 in, 2 out]
                }
                frame #31 {
                  n3607 = property on="data" class="Arr (strict)"() -> ("Value"=w4881:dbl[])  [unwired: 2 in, 2 out]
                  n3608 = property on="PT1" class="Bool (strict)"() -> ("Value"=w4880:bool)  [unwired: 2 in, 2 out]
                  n3609 = case shown="True" w4880 {
                    tunnel: w4881 -> [w4883 w4887]
                    tunnel: [w4883 w4886] -> w4882
                    frame False {
                      # "we are not Measuring magnetic field on IPS120-0"
                    }
                    frame True {
                      # "Measure  SH_T on Teslatron"
                      n3610 = call "TRITON_Read Temperature.vi"("Channel"=7 ("Ch2")) -> ("Measuremet"=w4884:dbl)  [unwired: 1 in, 1 out]
                      n3611 = Build Array (concatenate)(w4887, w4884) -> (w4886:dbl[])
                    }
                  }
                  n3612 = property on="data" class="Arr (strict)"("Value"=w4882) -> ()  [unwired: 2 in, 2 out]
                }
                frame #32 {
                  # "check if current \non 2461 SouceMeter\nis to be measured"
                  n3613 = property on="data" class="Arr (strict)"() -> ("Value"=w4889:dbl[])  [unwired: 2 in, 2 out]
                  n3614 = property on="MC_RuO2" class="Bool (strict)"() -> ("Value"=w4888:bool)  [unwired: 2 in, 2 out]
                  n3615 = case shown="True" w4888 {
                    tunnel: w4889 -> [w4891 w4895]
                    tunnel: [w4891 w4894] -> w4890
                    frame False {
                      # "we are not measuring 2461, voltage (2461_meas_v)"
                    }
                    frame True {
                      # "we are  measuring 2461, voltage (2461_meas_v)"
                      n3616 = call "TRITON_Read Temperature.vi"("Channel"=8 ("Ch2")) -> ("Measuremet"=w4892:dbl)  [unwired: 1 in, 1 out]
                      n3617 = Build Array (concatenate)(w4895, w4892) -> (w4894:dbl[])
                    }
                  }
                  n3618 = property on="data" class="Arr (strict)"("Value"=w4890) -> ()  [unwired: 2 in, 2 out]
                }
                frame #33 {
                  # "check if current \non 2461 SouceMeter\nis to be measured"
                  n3619 = property on="data" class="Arr (strict)"() -> ("Value"=w4897:dbl[])  [unwired: 2 in, 2 out]
                  n3620 = property on="Still" class="Bool (strict)"() -> ("Value"=w4896:bool)  [unwired: 2 in, 2 out]
                  n3621 = case shown="True" w4896 {
                    tunnel: w4897 -> [w4899 w4903]
                    tunnel: [w4899 w4902] -> w4898
                    frame False {
                      # "we are not measuring 2461, voltage (2461_meas_v)"
                    }
                    frame True {
                      # "we are  measuring 2461, voltage (2461_meas_v)"
                      n3622 = call "TRITON_Read Temperature.vi"("Channel"=3 ("Ch2")) -> ("Measuremet"=w4900:dbl)  [unwired: 1 in, 1 out]
                      n3623 = Build Array (concatenate)(w4903, w4900) -> (w4902:dbl[])
                    }
                  }
                  n3624 = property on="data" class="Arr (strict)"("Value"=w4898) -> ()  [unwired: 2 in, 2 out]
                }
                frame #34 {
                  # "check if current \non 2461 SouceMeter\nis to be measured"
                  n3625 = property on="data" class="Arr (strict)"() -> ("Value"=w4905:dbl[])  [unwired: 2 in, 2 out]
                  n3626 = property on="Cold_Plate" class="Bool (strict)"() -> ("Value"=w4904:bool)  [unwired: 2 in, 2 out]
                  n3627 = case shown="True" w4904 {
                    tunnel: w4905 -> [w4907 w4911]
                    tunnel: [w4907 w4910] -> w4906
                    frame False {
                      # "we are not measuring 2461, voltage (2461_meas_v)"
                    }
                    frame True {
                      # "we are  measuring 2461, voltage (2461_meas_v)"
                      n3628 = call "TRITON_Read Temperature.vi"("Channel"=4 ("Ch2")) -> ("Measuremet"=w4908:dbl)  [unwired: 1 in, 1 out]
                      n3629 = Build Array (concatenate)(w4911, w4908) -> (w4910:dbl[])
                    }
                  }
                  n3630 = property on="data" class="Arr (strict)"("Value"=w4906) -> ()  [unwired: 2 in, 2 out]
                }
                frame #35 {
                  # "check if current \non 2461 SouceMeter\nis to be measured"
                  n3631 = property on="data" class="Arr (strict)"() -> ("Value"=w4913:dbl[])  [unwired: 2 in, 2 out]
                  n3632 = property on="PT2" class="Bool (strict)"() -> ("Value"=w4912:bool)  [unwired: 2 in, 2 out]
                  n3633 = case shown="True" w4912 {
                    tunnel: w4913 -> [w4915 w4919]
                    tunnel: [w4915 w4918] -> w4914
                    frame False {
                      # "we are not measuring 2461, voltage (2461_meas_v)"
                    }
                    frame True {
                      # "we are  measuring 2461, voltage (2461_meas_v)"
                      n3634 = call "TRITON_Read Temperature.vi"("Channel"=2 ("Ch2")) -> ("Measuremet"=w4916:dbl)  [unwired: 1 in, 1 out]
                      n3635 = Build Array (concatenate)(w4919, w4916) -> (w4918:dbl[])
                    }
                  }
                  n3636 = property on="data" class="Arr (strict)"("Value"=w4914) -> ()  [unwired: 2 in, 2 out]
                }
                frame #36 {
                  # "check if current \non 2461 SouceMeter\nis to be measured"
                  n3637 = property on="data" class="Arr (strict)"() -> ("Value"=w4921:dbl[])  [unwired: 2 in, 2 out]
                  n3638 = property on="MC_Cernox" class="Bool (strict)"() -> ("Value"=w4920:bool)  [unwired: 2 in, 2 out]
                  n3639 = case shown="True" w4920 {
                    tunnel: w4921 -> [w4923 w4927]
                    tunnel: [w4923 w4926] -> w4922
                    frame False {
                      # "we are not measuring 2461, voltage (2461_meas_v)"
                    }
                    frame True {
                      # "we are  measuring 2461, voltage (2461_meas_v)"
                      n3640 = call "TRITON_Read Temperature.vi"("Channel"=5 ("Ch2")) -> ("Measuremet"=w4924:dbl)  [unwired: 1 in, 1 out]
                      n3641 = Build Array (concatenate)(w4927, w4924) -> (w4926:dbl[])
                    }
                  }
                  n3642 = property on="data" class="Arr (strict)"("Value"=w4922) -> ()  [unwired: 2 in, 2 out]
                }
                frame #37 {
                  # "check if current \non 2461 SouceMeter\nis to be measured"
                  n3643 = property on="2461_meas_v" class="Bool (strict)"() -> ("Value"=w4928:bool)  [unwired: 2 in, 2 out]
                  n3644 = property on="data" class="Arr (strict)"() -> ("Value"=w4929:dbl[])  [unwired: 2 in, 2 out]
                  n3645 = case shown="True" w4928 {
                    tunnel: w4929 -> [w4931 w4936]
                    tunnel: [w4931 w4935] -> w4930
                    frame False {
                      # "we are not measuring 2461, voltage (2461_meas_v)"
                    }
                    frame True {
                      # "we are  measuring 2461, voltage (2461_meas_v)"
                      n3646 = property on="2461_addr_sweep" class="VISAName"() -> ("Value"=w4933:refnum<visa-resource-name>)  [unwired: 2 in, 2 out]
                      n3647 = call <instrlib>:"Read (Single Point).vi"("VISA resource name"=w4933) -> ("Data out"=w4932:string)  [unwired: 12 in, 2 out]
                      n3648 = Fract/Exp String To Number(string=w4932) -> (number=w4934:dbl)  [unwired: 3 in, 1 out]
                      n3649 = Build Array (concatenate)(w4936, w4934) -> (w4935:dbl[])
                    }
                  }
                  n3650 = property on="data" class="Arr (strict)"("Value"=w4930) -> ()  [unwired: 2 in, 2 out]
                }
                frame #38 {
                  # "check if current \non 2461 SouceMeter\nis to be measured"
                  n3651 = property on="2461_meas_i" class="Bool (strict)"() -> ("Value"=w4937:bool)  [unwired: 2 in, 2 out]
                  n3652 = property on="data" class="Arr (strict)"() -> ("Value"=w4938:dbl[])  [unwired: 2 in, 2 out]
                  n3653 = case shown="True" w4937 {
                    tunnel: w4938 -> [w4940 w4944]
                    tunnel: [w4940 w4943] -> w4939
                    frame False {
                      # "we are not measuring 2461, voltage (2461_meas_v)"
                    }
                    frame True {
                      # "we are  measuring 2461, curent (2461_meas_i)"
                      n3654 = property on="2461_addr_sweep" class="VISAName"() -> ("Value"=w4942:refnum<visa-resource-name>)  [unwired: 2 in, 2 out]
                      n3655 = call <instrlib>:"Get Source Level.vi"("VISA resource name"=w4942) -> ("Current Level Out"=w4941:dbl)  [unwired: 7 in, 3 out]
                      n3656 = Build Array (concatenate)(w4944, w4941) -> (w4943:dbl[])
                    }
                  }
                  n3657 = property on="data" class="Arr (strict)"("Value"=w4939) -> ()  [unwired: 2 in, 2 out]
                }
                frame #39 {
                  # "Measure MFLI_V if \nit is checked"
                  n3658 = property on="MFLI1_d0" class="Bool (strict)"() -> ("Value"=w4945:bool)  [unwired: 2 in, 2 out]
                  n3659 = property on="data" class="Arr (strict)"() -> ("Value"=w4947:dbl[])  [unwired: 2 in, 2 out]
                  n3660 = case shown="True" w4945 {
                    tunnel: w4947 -> [w4948 w4953]
                    tunnel: [w4948 w4952] -> w4946
                    frame False {
                      # "We are not recording Step Value if it is linetrace"
                    }
                    frame True {
                      n3661 = flat-sequence {
                        tunnel: [w4957] -> w4951
                        tunnel: [w4956] -> w4950
                        tunnel: [w4955] -> w4949
                        frame #0 {
                          n3662 = property on="HandleOut" class="Clust (strict)"() -> ("Value"=w4959:T1)  [unwired: 2 in, 2 out]
                          n3663 = call "MFLIcontrol.vi"("MFLI function"=MFLIcommand."measure XY on demod0", "handle in"=w4959) -> ("Demod Sample Out 2"=w4954:T20)  [unwired: 5 in, 4 out]
                          n3664 = Unbundle(w4954) -> ("X (Vrms)"=w4957:dbl, "Y (Vrms)"=w4956:dbl, "Freq (Hz)"=w4955:dbl)  [unwired: 6 out]
                        }
                      }
                      n3665 = Build Array (concatenate)(w4953, w4951, w4950, w4949) -> (w4952:dbl[])
                    }
                  }
                  n3666 = property on="data" class="Arr (strict)"("Value"=w4946) -> ()  [unwired: 2 in, 2 out]
                }
                frame #40 {
                  # "Measure MFLI_V if \nit is checked"
                  n3667 = property on="MFLI1_d1" class="Bool (strict)"() -> ("Value"=w4960:bool)  [unwired: 2 in, 2 out]
                  n3668 = property on="data" class="Arr (strict)"() -> ("Value"=w4962:dbl[])  [unwired: 2 in, 2 out]
                  n3669 = case shown="True" w4960 {
                    tunnel: w4962 -> [w4963 w4968]
                    tunnel: [w4963 w4967] -> w4961
                    frame False {
                      # "We are not recording Step Value if it is linetrace"
                    }
                    frame True {
                      n3670 = flat-sequence {
                        tunnel: [w4972] -> w4966
                        tunnel: [w4971] -> w4965
                        tunnel: [w4970] -> w4964
                        frame #0 {
                          n3671 = property on="HandleOut" class="Clust (strict)"() -> ("Value"=w4974:T1)  [unwired: 2 in, 2 out]
                          n3672 = call "MFLIcontrol.vi"("MFLI function"=MFLIcommand."measure XY on demod1", "handle in"=w4974) -> ("Demod Sample Out 2"=w4969:T20)  [unwired: 5 in, 4 out]
                          n3673 = Unbundle(w4969) -> ("X (Vrms)"=w4972:dbl, "Y (Vrms)"=w4971:dbl, "Freq (Hz)"=w4970:dbl)  [unwired: 6 out]
                        }
                      }
                      n3674 = Build Array (concatenate)(w4968, w4966, w4965, w4964) -> (w4967:dbl[])
                    }
                  }
                  n3675 = property on="data" class="Arr (strict)"("Value"=w4961) -> ()  [unwired: 2 in, 2 out]
                }
                frame #41 {
                  # "Measure MFLI_V if \nit is checked"
                  n3676 = property on="MFLI1_d2" class="Bool (strict)"() -> ("Value"=w4975:bool)  [unwired: 2 in, 2 out]
                  n3677 = property on="data" class="Arr (strict)"() -> ("Value"=w4977:dbl[])  [unwired: 2 in, 2 out]
                  n3678 = case shown="True" w4975 {
                    tunnel: w4977 -> [w4978 w4983]
                    tunnel: [w4978 w4982] -> w4976
                    frame False {
                      # "We are not recording Step Value if it is linetrace"
